vi "Log Error.vi"(8 "error in (no error)":errorcluster, 10 "LabActor Error":T1, 11 "Error Log in":refnum<class "Error Log.lvclass">) -> (0 "error out":errorcluster, 3 "Error Log out":refnum<class "Error Log.lvclass">)   [LabVIEW 2024, in "Error Log.lvclass"]
uses:
  Error Log.lvclass
  Template Module/LabActor Error.ctl
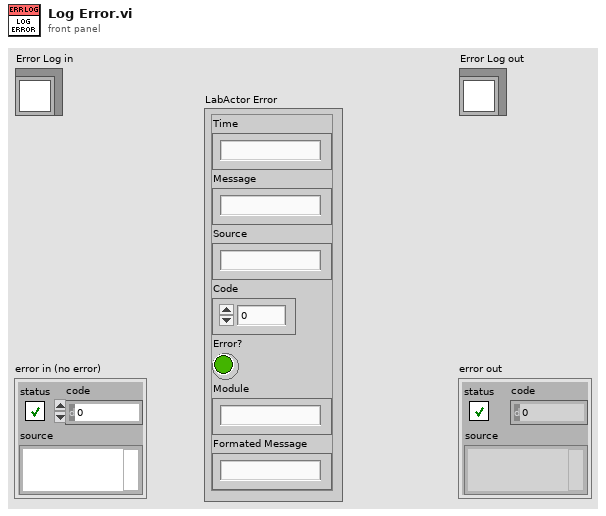
[diagram p1: front panel]
types:
  T1 = typedef "LabActor Error.ctl" = cluster{"Time":string, "Message":string, "Source":string, "Code":i32, "Error?":bool, "Module":string, "Formated Message":string}
  T2 = enum16{"open", "replace", "create", "open or create", "replace or create", "replace or create with confirmation"}
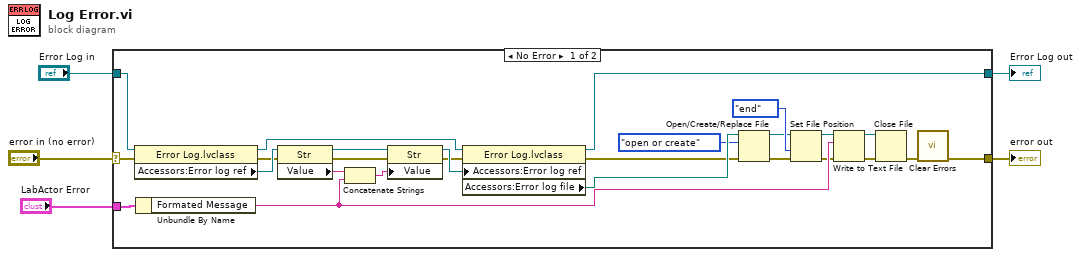
[diagram p0: block diagram]
diagram:
  n1 = case shown="No Error" "error in (no error)" {
    selector: "error in (no error)" -> [w31 w33]
    tunnel: [w17 w33] -> w4
    tunnel: [w19 w32] -> w2
    tunnel: "Error Log in" -> [w30 w32]
    tunnel: "LabActor Error" -> [w25 _]
    frame No Error {
      n2 = property class="Error Log.lvclass"(reference=w30, error in=w31) -> (reference out=w23:refnum<class "Error Log.lvclass">, error out=w28:errorcluster, "Accessors:Error log ref"=w29:refnum<vi>)
      n3 = Unbundle By Name(w25) -> ("Formated Message"=w18:string)
      n4 = property class="Str"(reference=w29, error in=w28) -> (reference out=w27:refnum<vi>, error out=w21:errorcluster, "Value"=w26:string)
      n5 = Concatenate Strings(w26, w18) -> (w24:string)
      n6 = property class="Str"(reference=w27, error in=w21, "Value"=w24) -> (reference out=w22:refnum<vi>, error out=w20:errorcluster)
      n7 = property class="Error Log.lvclass"(reference=w23, error in=w20, "Accessors:Error log ref"=w22) -> (reference out=w19:refnum<class "Error Log.lvclass">, error out=w15:errorcluster, "Accessors:Error log file"=w16:path)
      n8 = Open/Create/Replace File(file path (use dialog)=w16, error in=w15, operation (0:open)=T2."open or create") -> (refnum out=w8:refnum<file>, error out=w7:errorcluster)  [unwired: 3 in, 1 out]
      n9 = Set File Position(refnum=w8, from (0:start)=enum16{"start", "end", "current"}."end", error in=w7) -> (refnum out=w12:refnum<file>, error out=w13:errorcluster)  [unwired: 1 in]
      n10 = Write to Text File(file (use dialog)=w12, text=w18, error in=w13) -> (refnum out=w11:refnum<file>, error out=w10:errorcluster)  [unwired: 1 in, 1 out]
      n11 = Close File(refnum=w11, error in=w10) -> (error out=w9:errorcluster)  [unwired: 1 out]
      n12 = call <vilib>:"Clear Errors.vi"("error in (no error)"=w9) -> ("error out"=w17:errorcluster)  [unwired: 5 in, 1 out]
    }
    frame Error {
    }
  }
  "error out" <- w4
  "Error Log out" <- w2
